vi "BallWithVelocityDestModifier.vi"(7 "destino original":dbl[](array[numeric]), 8 "error in (no error)":errorcluster, 9 "Robot in":refnum<class "Robot.lvclass">, 10 "Game":refnum<class "Game.lvclass">, 11 "KickToSkill in":refnum<class "KickToSkill.lvclass">) -> (0 "error out":errorcluster, 2 "destino com velocidade":dbl[](array[numeric]), 3 "KickToSkill out":refnum<class "KickToSkill.lvclass">)   [LabVIEW 2021, in "KickToSkill.lvclass"]
uses:
  KickToSkill.lvclass
  Game_class/Game.lvclass
  Robot_class/Robot.lvclass
  D:/RoboIme/horie/SSL_AI/Object_class/Object.lvclass
  Game_class/Game.lvclass/Game.ctl
  Ball_class/Ball.lvclass/Ball.ctl
  Object_class/Object.lvclass/Object.ctl
  Robot_class/Robot.lvclass/Robot.ctl
  <vilib>/Analysis/baseanly.llb/Unit Vector (DBL).vi
  Object_class/Read position(x,y).vi
  Robot_class/Read est_v_tang.vi
  Robot_class/Read est_v_norm.vi
  Game_class/Read BallRef.vi
  Ball_class/Read v_x.vi
  Ball_class/Read v_y.vi
  Ball_class/Ball.lvclass
  <vilib>/Analysis/NI_AALBase.lvlib
  <vilib>/Analysis/baseanly.llb/Real Dot Product.vi
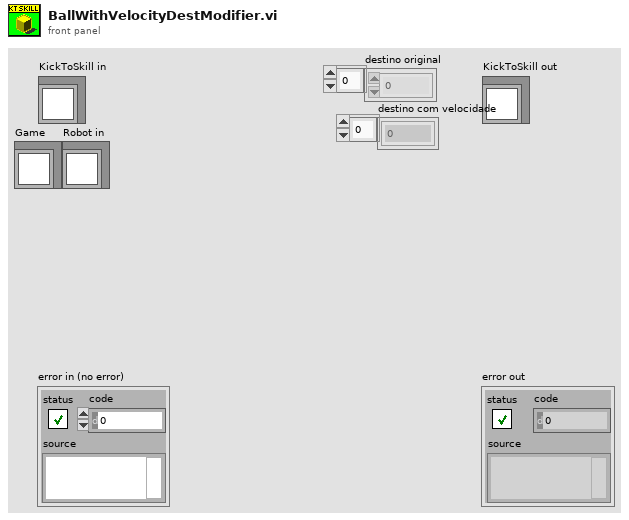
[diagram p1: front panel]
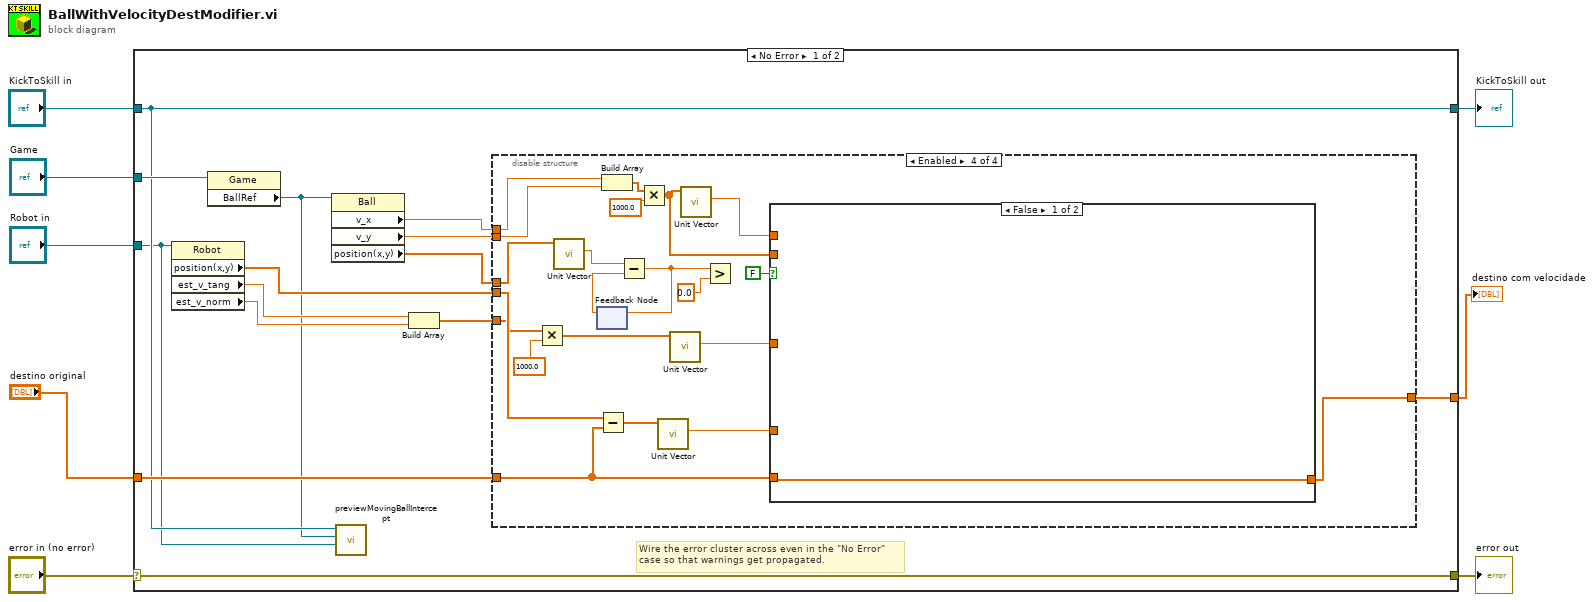
[diagram p0: block diagram]
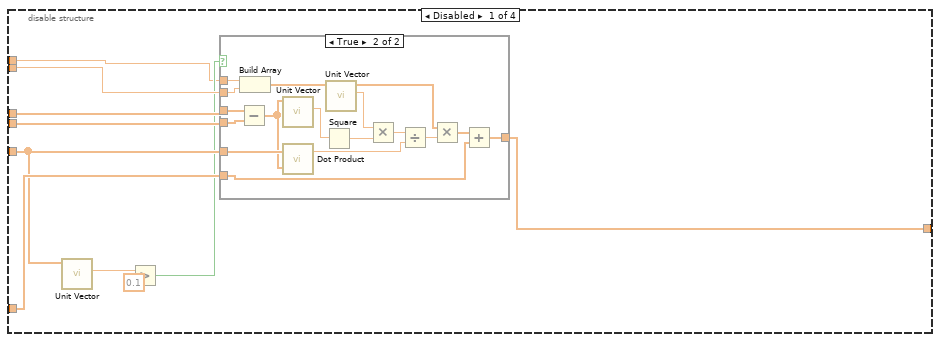
[diagram p2: hidden frame]
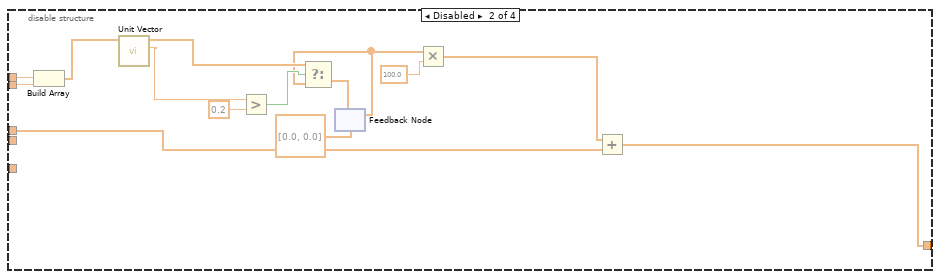
[diagram p4: hidden frame]
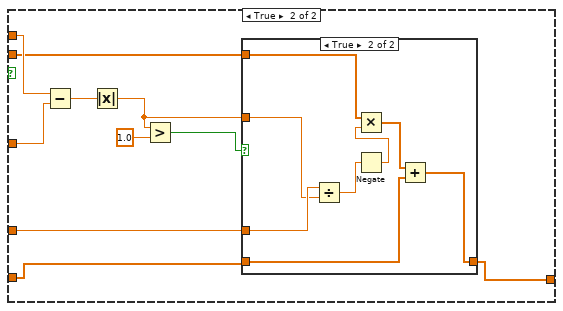
[diagram p6: hidden frame]
diagram:
  n1 = case shown="No Error" "error in (no error)" {
    selector: "error in (no error)" -> [w22 w109]
    tunnel: [w22 w109] -> w7
    tunnel: [w12 w108] -> w5
    tunnel: "KickToSkill in" -> [w12 w108]
    tunnel: "Game" -> [w21 _]
    tunnel: "Robot in" -> [w11 _]
    tunnel: "destino original" -> [w15 w107]
    tunnel: [w9 w107] -> w1
    frame No Error {
      # "Wire the error cluster across even in the \"No Error\"\ncase so that warnings get propagated."
      n2 = property class="Robot"(reference=w11) -> ("position(x,y)"=w18:dbl[], "est_v_tang"=w17:dbl, "est_v_norm"=w16:dbl)  [unwired: 1 in, 2 out]
      n3 = property class="Game"(reference=w21) -> ("BallRef"=w10:refnum<class "Ball.lvclass">)  [unwired: 1 in, 2 out]
      n4 = property class="Ball"(reference=w10) -> ("v_x"=w13:dbl, "v_y"=w20:dbl, "position(x,y)"=w19:dbl[])  [unwired: 1 in, 2 out]
      n5 = call "previewMovingBallIntercept.vi"("Robot in"=w11, "BallRef"=w10, "KickToSkill in"=w12) -> ()  [unwired: 5 in, 4 out]
      n6 = Build Array(w17, w16) -> (w14:dbl[])
      n7 = disable-structure shown="Enabled" {
        disable-tunnel: w20 -> [w32 w63 _ w76]
        disable-tunnel: w19 -> [w31 w62 _ w86]
        disable-tunnel: w18 -> [w30 _ _ w80]
        disable-tunnel: w15 -> [w29 _ w65 w79]
        disable-tunnel: [w28 w61 w65 w81] -> w9
        disable-tunnel: w14 -> [w27 _ _ w69]
        disable-tunnel: w13 -> [w23 w64 _ w77]
        frame Disabled {
          n8 = call-poly <vilib>:"Unit Vector.vi"("Input Vector"=w27) -> ("norm"=w26:dbl)  [unwired: 8 in, 2 out]
          n9 = Greater?(x=w26, y=0.1) -> (0:w24:bool)
          n10 = case shown="True" w24 {
            tunnel: w23 -> [_ w50]
            tunnel: w32 -> [_ w49]
            tunnel: w31 -> [_ w48]
            tunnel: w30 -> [_ w46]
            tunnel: w29 -> [w33 w40]
            tunnel: [w33 w39] -> w28
            tunnel: w27 -> [_ w36]
            frame False {
            }
            frame True {
              n11 = Subtract(x=w48, y=w46) -> (x-y=w35:dbl[])
              n12 = Build Array(w50, w49) -> (w47:dbl[])
              n13 = call-poly <vilib>:"Unit Vector.vi"("Input Vector"=w35) -> ("norm"=w38:dbl)  [unwired: 8 in, 2 out]
              n14 = call-poly <vilib>:"Dot Product.vi"("Y Vector"=w35, "X Vector"=w36) -> ("X * Y"=w34:dbl)  [unwired: 1 out]
              n15 = Square(x=w38) -> (x^2=w37:dbl)
              n16 = call-poly <vilib>:"Unit Vector.vi"("Input Vector"=w47) -> ("norm"=w45:dbl, "Unit Vector"=w43:dbl[])  [unwired: 8 in, 1 out]
              n17 = Multiply(x=w45, y=w37) -> (x*y=w44:dbl)
              n18 = Divide(x=w44, y=w34) -> (x/y=w42:dbl)
              n19 = Multiply(x=w43, y=w42) -> (x*y=w41:dbl[])
              n20 = Add(x=w41, y=w40) -> (x+y=w39:dbl[])
            }
          }
        }
        frame Disabled {
          n21 = Build Array(w64, w63) -> (w60:dbl[])
          n22 = call-poly <vilib>:"Unit Vector.vi"("Input Vector"=w60) -> ("norm"=w58:dbl, "Unit Vector"=w55:dbl[])  [unwired: 8 in, 1 out]
          n23 = Greater?(x=w58, y=0.2) -> (0:w56:bool)
          n24 = feedback #1(dbl[] [0.0, 0.0] ("Unit Vector")) -> (w53:dbl[])
          n25 = Select(t=w55, s=w56, f=w53) -> (s? t:f=w54:dbl[])
          n26 = feedback-in #1(w54) -> ()
          n27 = Multiply(x=w53, y=100.0) -> (x*y=w52:dbl[])
          n28 = Add(x=w52, y=w62) -> (x+y=w61:dbl[])
        }
        frame Disabled {
        }
        frame Enabled {
          n29 = Multiply(x=w69, y=1000.0) -> (x*y=w67:dbl[])
          n30 = call-poly <vilib>:"Unit Vector.vi"("Input Vector"=w86) -> ("norm"=w85:dbl)  [unwired: 8 in, 2 out]
          n31 = feedback #2() -> (w84:dbl)  [unwired: 1 in]
          n32 = Subtract(x=w80, y=w79) -> (x-y=w78:dbl[])
          n33 = Build Array(w77, w76) -> (w72:dbl[])
          n34 = Subtract(x=w85, y=w84) -> (x-y=w83:dbl)
          n35 = feedback-in #2(w83) -> ()
          n36 = Multiply(x=w72, y=1000.0) -> (x*y=w70:dbl[])
          n37 = call-poly <vilib>:"Unit Vector.vi"("Input Vector"=w78) -> ("norm"=w73:dbl)  [unwired: 8 in, 2 out]
          n38 = call-poly <vilib>:"Unit Vector.vi"("Input Vector"=w67) -> ("norm"=w74:dbl)  [unwired: 8 in, 2 out]
          n39 = call-poly <vilib>:"Unit Vector.vi"("Input Vector"=w70) -> ("norm"=w75:dbl)  [unwired: 8 in, 2 out]
          n40 = Greater?(x=w83, y=0.0) -> ()  [unwired: 1 out]
          n41 = case shown="False" FALSE {
            tunnel: w79 -> [w87 w92]
            tunnel: [w87 w91] -> w81
            tunnel: w75 -> [_ w97]
            tunnel: w74 -> [_ w96]
            tunnel: w73 -> [_ w90]
            tunnel: w70 -> [_ w88]
            frame False {
            }
            frame True {
              n42 = Subtract(x=w97, y=w96) -> (x-y=w95:dbl)
              n43 = Absolute Value(x=w95) -> (abs(x)=w89:dbl)
              n44 = Greater?(x=w89, y=1.0) -> (0:w93:bool)
              n45 = case shown="True" w93 {
                tunnel: w92 -> [w98 w102]
                tunnel: [w98 w101] -> w91
                tunnel: w90 -> [_ w106]
                tunnel: w89 -> [_ w105]
                tunnel: w88 -> [_ w104]
                frame False {
                }
                frame True {
                  n46 = Divide(x=w106, y=w105) -> (x/y=w100:dbl)
                  n47 = Negate(x=w100) -> (-x=w99:dbl)
                  n48 = Multiply(x=w104, y=w99) -> (x*y=w103:dbl[])
                  n49 = Add(x=w103, y=w102) -> (x+y=w101:dbl[])
                }
              }
            }
          }
        }
      }
    }
    frame Error {
    }
  }
  "error out" <- w7
  "KickToSkill out" <- w5
  "destino com velocidade" <- w1
